vi "Write Bounds.vi"(3 "(FPSZ)":refnum<class "FPSZ.lvclass">, 4 "Bounds":T1) -> (5 "(FPSZ) Out":refnum<class "FPSZ.lvclass">)   [LabVIEW 2020, in "FPSZ.lvclass"]
uses:
  FPSZ.lvclass
  <vilib>/Utility/miscctls.llb/LVBoundsTypeDef.ctl
  FPSZ.lvclass/FPSZ.ctl
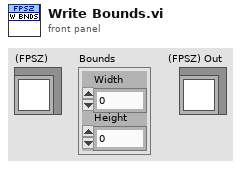
[diagram p1: front panel]
types:
  T1 = typedef "LVBoundsTypeDef.ctl" = cluster{"Width":u32, "Height":u32}
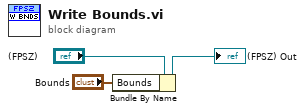
[diagram p0: block diagram]
diagram:
  n1 = Bundle By Name(cluster="(FPSZ)", "Bounds"="Bounds") -> (→"(FPSZ) Out":refnum<class "FPSZ.lvclass">)
